vi "grabber tracking display panel.vi"() -> ()   [LabVIEW 2010]
uses:
  internal_queues.ctl
  line_info.ctl
  volume_with_lines.ctl
  volume_info.ctl
  kalman_result_scaled.ctl
  location3D.ctl
  spot location.ctl
panel:
  in  "Queues":T1
  in  "pos history time":dbl=10.0
  in  "photon history time":dbl=60.0
  in  "photon graph type":enum16{"red", "green", "ratio"}(ring)
  out "file access error":bool
  out "tracking":bool
  in  "stop":bool
  in  "purge history":bool
  in  "close file":bool
  in  "open file for writing":bool
  out "photons":cluster{"t":dbl[], "x":dbl[]}[](graph)
  out "position":cluster{"t":dbl[], "x":dbl[]}[](graph)
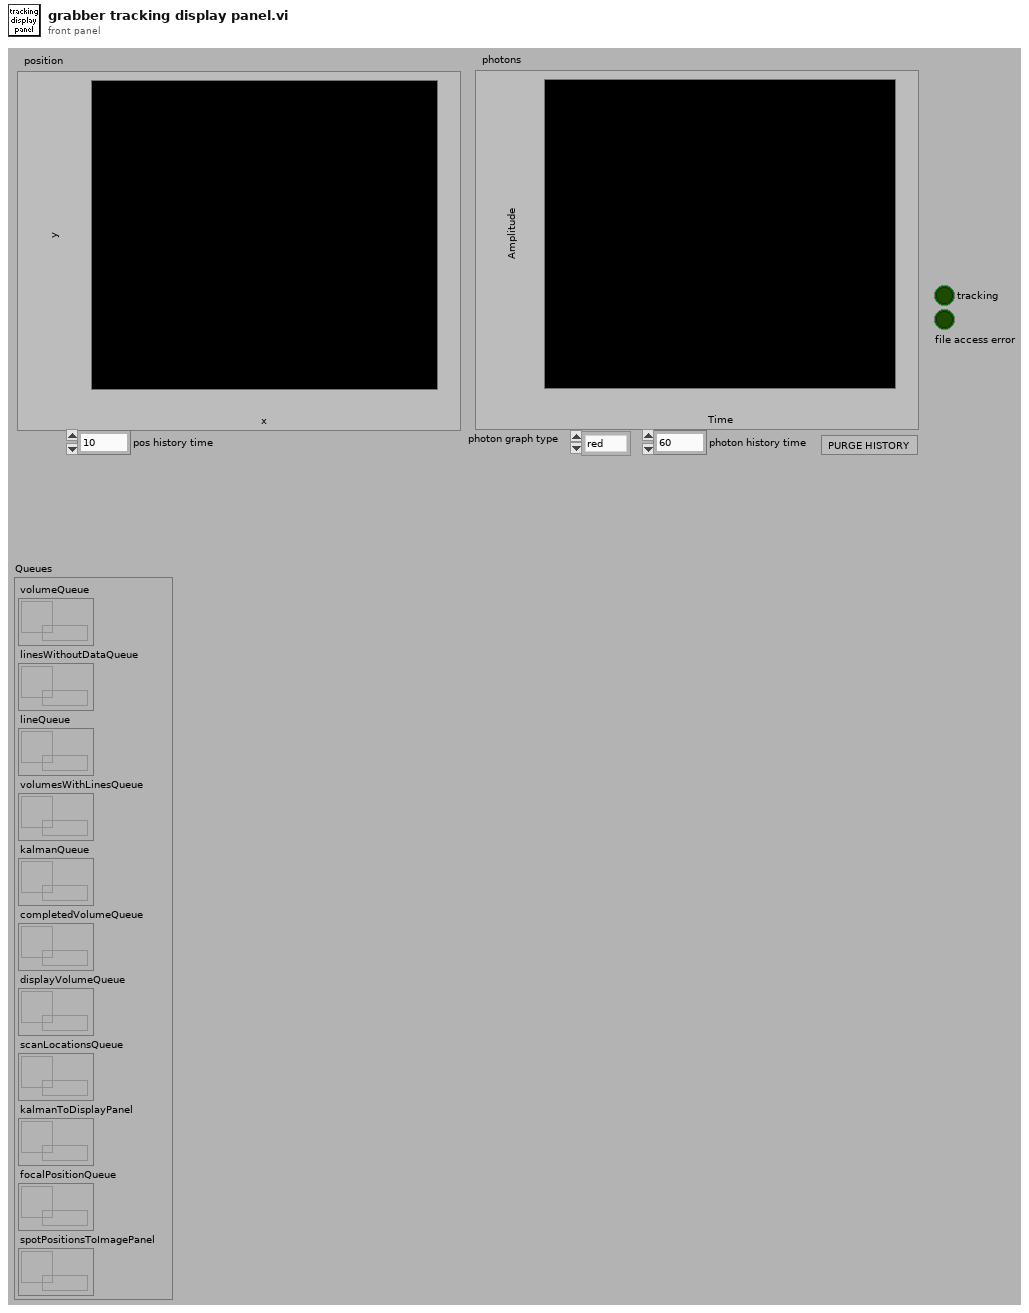
[diagram p1: front panel]
types:
  T1 = typedef "internal_queues.ctl" = cluster{"volumeQueue":refnum<queue>, "linesWithoutDataQueue":refnum<queue>, "lineQueue":refnum<queue>, "volumesWithLinesQueue":refnum<queue>, "kalmanQueue":refnum<queue>, "completedVolumeQueue":refnum<queue>, "displayVolumeQueue":refnum<queue>, "scanLocationsQueue":refnum<queue>, "kalmanToDisplayPanel":refnum<queue>, "focalPositionQueue":refnum<queue>, "spotPositionsToImagePanel":refnum<queue>}
  T2 = cluster{"pos":cluster{"weighted sum":dbl, "n measurements":dbl, "t values":dbl[], "x values":dbl[], "t start":dbl}[], "red":cluster{"weighted sum":dbl, "n measurements":dbl, "t values":dbl[], "x values":dbl[], "t start":dbl}, "green":cluster{"weighted sum":dbl, "n measurements":dbl, "t values":dbl[], "x values":dbl[], "t start":dbl}, "ratio":cluster{"weighted sum":dbl, "n measurements":dbl, "t values":dbl[], "x values":dbl[], "t start":dbl}, "SPPF state":cluster{"theta":dbl[], "w":dbl[][], "elapsed time":dbl}}[]
  T3 = typedef "kalman_result_scaled.ctl" = cluster{"axis":u8, "pos":dbl, "vel":dbl, "p_err":dbl, "status":u32, "n photon ch 0":u32, "n photon ch 1":u32, "elapsed time":dbl}
  T4 = enum16{"open", "replace", "create", "open or create", "replace or create", "replace or create with confirmation"}
  T5 = typedef "spot location.ctl" = cluster{"x (um)":dbl, "y (um)":dbl, "z (um)":dbl, "spot number":u8}
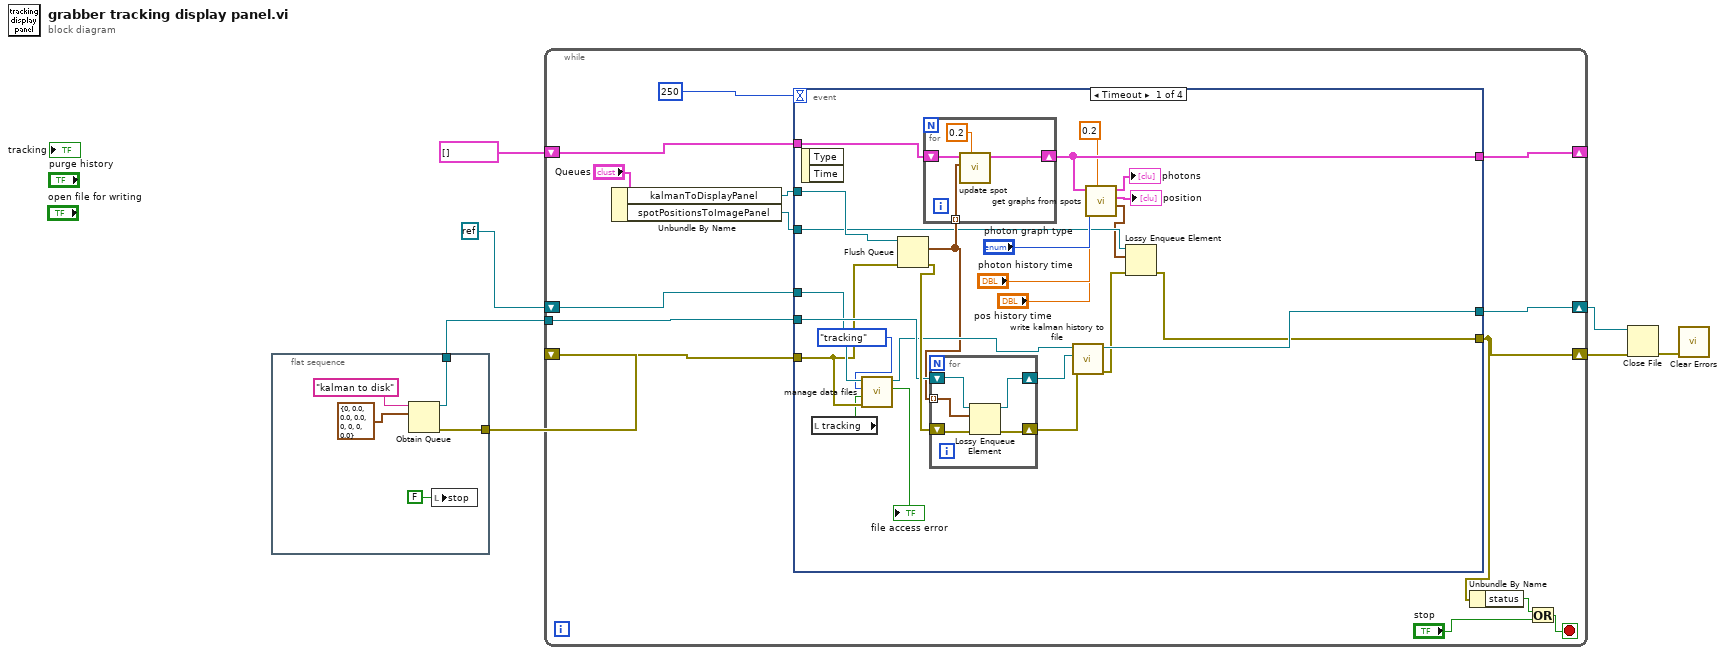
[diagram p0: block diagram]
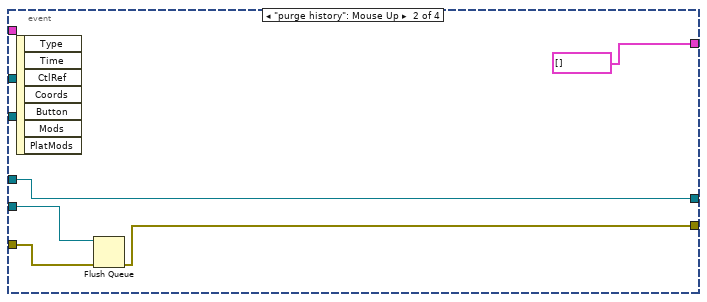
[diagram p2: hidden frame]
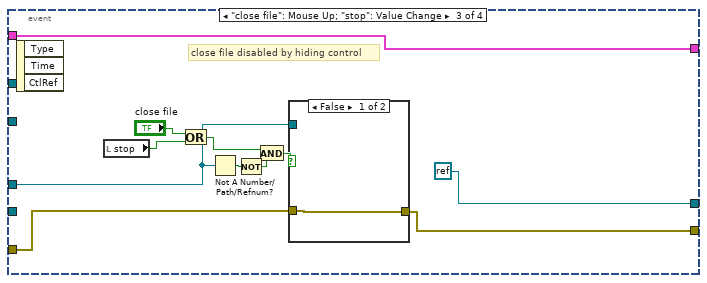
[diagram p3: hidden frame]
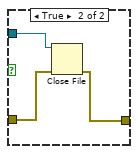
[diagram p4: hidden frame]
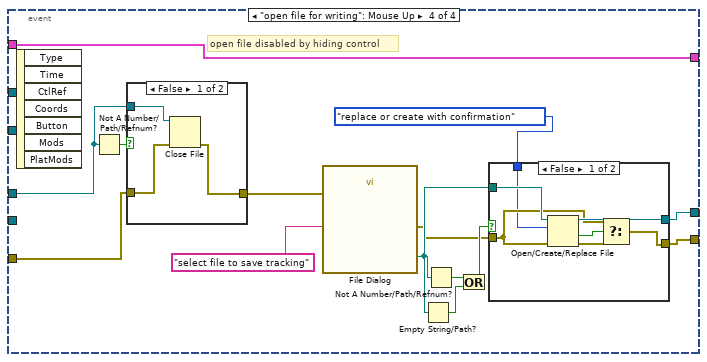
[diagram p5: hidden frame]
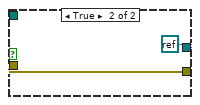
[diagram p7: hidden frame]
diagram:
  n1 = flat-sequence {
    tunnel: [w10] -> w7
    tunnel: [w9] -> w6
    frame #0 {
      n2 = Obtain Queue(name (unnamed)="kalman to disk", element data type=T3 {"axis"=0, "pos"=0.0, "vel"=0.0, "p_err"=0.0, "status"=0, "n photon ch 0"=0, "n photon ch 1"=0, "elapsed time"=0.0} ("element")) -> (queue out=w10:refnum<queue>, error out=w9:errorcluster)  [unwired: 3 in, 1 out]
      n3 = local write "stop"(FALSE ("stop")) -> ()
    }
  }
  n4 = while {
    shift-right: [w21] -> w4
    shift-left: w6 -> [w25]
    shift-right: [w24] -> w3
    shift-left: refnum<k0> refnum -> [w23]
    tunnel: w7 -> [w22]
    shift-right: [w17] -> _
    shift-left: T2 [] ("spots out") -> [w16]
    stop <- w19 stop-if-true
    n5 = Unbundle By Name("Queues") -> ("kalmanToDisplayPanel"=w14:refnum<queue>, "spotPositionsToImagePanel"=w13:refnum<queue>)
    n6 = event shown="[0] Timeout" {
      selector: _ -> [_ _ _ _]
      dyn-events: _ -> [_ _ _ _]
      timeout: 250 -> [_ _ _ _]
      tunnel: w25 -> [w44 w65 w76 w85]
      tunnel: [w27 w63 w75 w88] -> w21
      tunnel: [w48 w62 refnum<k0> refnum w87] -> w24
      tunnel: w23 -> [w46 w62 w73 w86]
      tunnel: w22 -> [w47 w64 _ _]
      tunnel: [w38 T2 [] ("spots out") w66 w81] -> w17
      tunnel: w16 -> [w40 _ w66 w81]
      tunnel: w14 -> [w31 _ _ _]
      tunnel: w13 -> [w30 _ _ _]
      event Timeout {
        n7 = event-data() -> ()  [unwired: 1 in, 2 out]
        n8 = local read "tracking"() -> (w42:bool)
        n9 = call "manage data files.vi"("error in"=w44, "tracking"=w42, "recording type"=enum16{"tracking", "stage"}."tracking", "refnum in"=w46) -> ("file access error"=→"file access error":bool, "refnum out"=w45:refnum<file>)  [unwired: 4 in, 2 out]
        n10 = Flush Queue(queue=w31, error in (no error)=w44) -> (remaining elements=w39:T3[], error out=w51:errorcluster)  [unwired: 1 out]
        n11 = for {
          shift-right: [w55] -> w38
          shift-left: w40 -> [w54]
          tunnel: w39 -> [w53] mode=indexing
          n12 = call "update spot.vi"("dt"=0.2, "kalman result"=w53, "Spots"=w54) -> ("spots out"=w55:T2)  [unwired: 8 in]
        }
        n13 = for {
          tunnel: w39 -> [w58] mode=indexing
          shift-right: [w56] -> w49
          shift-left: w47 -> [w59]
          shift-right: [w57] -> w50
          shift-left: w51 -> [w60]
          n14 = Lossy Enqueue Element(queue=w59, element=w58, error in (no error)=w60) -> (queue out=w56:refnum<queue>, error out=w57:errorcluster)  [unwired: 2 out]
        }
        n15 = call "write kalman history to file.vi"("error in (no error)"=w50, "kalmanQueue for output"=w49, "refnum"=w45) -> ("error out"=w28:errorcluster, "refnum out"=w48:refnum<file>)  [unwired: 7 in]
        n16 = call "get graphs from spots.vi"("delta t"=0.2, "pos history time"="pos history time", "photon history time"="photon history time", "photon graph type"="photon graph type", "spots"=w38) -> ("spot locations"=w29:T5[], "position graphs"=→"position":cluster{"yi":dbl[], "yi":dbl[]}[], "photon graphs"=→"photons":cluster{"t values":dbl[], "x values":dbl[]}[])  [unwired: 4 in]
        n17 = Lossy Enqueue Element(queue=w30, element=w29, error in (no error)=w28) -> (error out=w27:errorcluster)  [unwired: 3 out]
      }
      event "purge history": Mouse Up {
        n18 = event-data() -> ()  [unwired: 1 in, 7 out]
        n19 = Flush Queue(queue=w64, error in (no error)=w65) -> (error out=w63:errorcluster)  [unwired: 2 out]
      }
      event "close file": Mouse Up; "stop": Value Change {
        # "close file disabled by hiding control"
        n20 = event-data() -> ()  [unwired: 1 in, 3 out]
        n21 = local read "stop"() -> (w70:bool)
        n22 = Or(x="close file", y=w70) -> (x .or. y?=w67:bool)
        n23 = Not A Number/Path/Refnum?(number/path/refnum=w73) -> (NaN/Path/Refnum?=w72:bool)
        n24 = Not(x=w72) -> (.not. x?=w68:bool)
        n25 = And(x=w67, y=w68) -> (x .and. y?=w69:bool)
        n26 = case shown="False" w69 {
          tunnel: w76 -> [w77 w80]
          tunnel: w73 -> [_ w79]
          tunnel: [w77 w78] -> w75
          frame False {
          }
          frame True {
            n27 = Close File(refnum=w79, error in=w80) -> (error out=w78:errorcluster)  [unwired: 1 out]
          }
        }
      }
      event "open file for writing": Mouse Up {
        # "open file disabled by hiding control"
        n28 = event-data() -> ()  [unwired: 1 in, 7 out]
        n29 = Not A Number/Path/Refnum?(number/path/refnum=w86) -> (NaN/Path/Refnum?=w82:bool)
        n30 = case shown="False" w82 {
          tunnel: w85 -> [w97 w98]
          tunnel: w86 -> [w96 _]
          tunnel: [w95 w98] -> w84
          frame False {
            n31 = Close File(refnum=w96, error in=w97) -> (error out=w95:errorcluster)  [unwired: 1 out]
          }
          frame True {
          }
        }
        n32 = call "File Dialog"("prompt"="select file to save tracking", "error in"=w84) -> ("selected path"=w91:path, "error out"=w89:errorcluster)  [unwired: 10 in, 2 out]
        n33 = Empty String/Path?(string/path=w91) -> (empty?=w92:bool)
        n34 = Not A Number/Path/Refnum?(number/path/refnum=w91) -> (NaN/Path/Refnum?=w93:bool)
        n35 = Or(x=w93, y=w92) -> (x .or. y?=w90:bool)
        n36 = case shown="False" w90 {
          tunnel: w91 -> [w105 _]
          tunnel: w89 -> [w100 w107]
          tunnel: [w101 w107] -> w88
          tunnel: [w104 refnum<k0> refnum] -> w87
          tunnel: T4."replace or create with confirmation" ("operation (0:open)") -> [w99 _]
          frame False {
            n37 = Open/Create/Replace File(file path (use dialog)=w105, error in=w100, operation (0:open)=w99) -> (refnum out=w104:refnum<file>, cancelled=w103:bool, error out=w102:errorcluster)  [unwired: 3 in]
            n38 = Select(t=w100, s=w103, f=w102) -> (s? t:f=w101:errorcluster)
          }
          frame True {
          }
        }
      }
    }
    n39 = Unbundle By Name(w21) -> ("status"=w20:bool)
    n40 = Or(x=w20, y="stop") -> (x .or. y?=w19:bool)
  }
  n41 = Close File(refnum=w3, error in=w4) -> (error out=w2:errorcluster)  [unwired: 1 out]
  n42 = call <vilib>:"Clear Errors.vi"("error in (no error)"=w2) -> ()  [unwired: 6 in, 1 out]
